vi "Deadzone.vi"(8 "error in (no error)":errorcluster, 10 "Deadzone":dbl, 11 "Input":dbl) -> (0 "error out":errorcluster, 2 "In deadzone?":bool, 3 "Output":dbl)   [LabVIEW 2014]
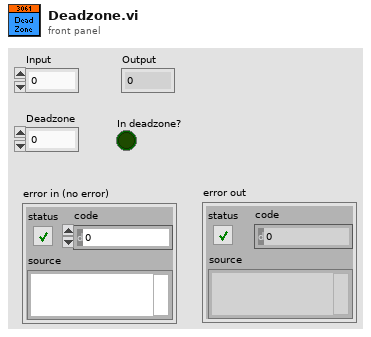
[diagram p1: front panel]
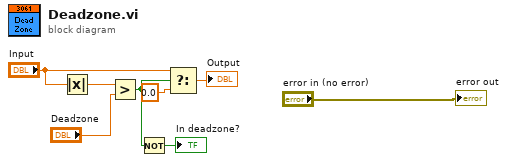
[diagram p0: block diagram]
diagram:
  n1 = Absolute Value(x="Input") -> (abs(x)=w7:dbl)
  n2 = Greater?(x=w7, y="Deadzone") -> (0:w6:bool)
  n3 = Not(x=w6) -> (.not. x?=→"In deadzone?":bool)
  n4 = Select(t="Input", s=w6, f=0.0) -> (s? t:f=→"Output":dbl)
  "error out" <- "error in (no error)"
